vi "Read Post-Setup Msgs.vi"(11 "Msg Self in":refnum<class "Msg Self.lvclass">) -> (2 "Post-Setup Msgs":refnum<class "Msg.lvclass">[](array[class]))   [LabVIEW 2020, in "jettl.lvlib" / "Msg Self.lvclass"]
uses:
  Msg Self.lvclass
  Msg/Msg.lvclass
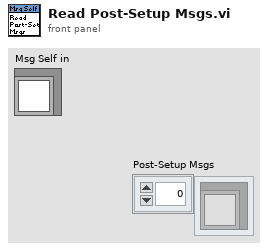
[diagram p1: front panel]
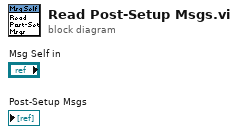
[diagram p0: block diagram]
diagram:
